vi "GlobalSavePathToStoreStack.vi"() -> ()   [LabVIEW 2011]
panel:
  in  "SaveStackPath":path
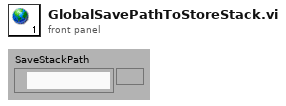
[diagram p1: front panel]
diagram:
